vi "InitImgPath.vi"(8 "error in":errorcluster, 10 "ConfigFilePath":path, 11 "Instance":i32) -> (0 "error out":errorcluster, 2 "ImgPath":path)   [LabVIEW 2016]
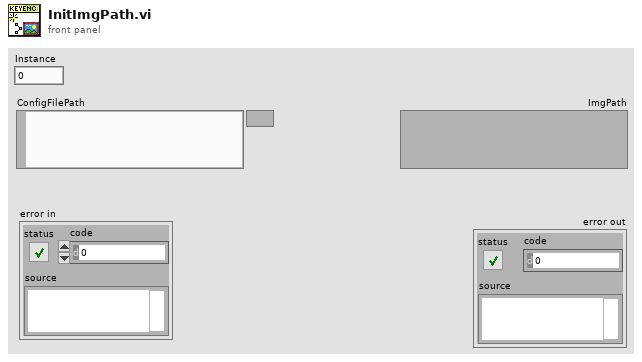
[diagram p1: front panel]
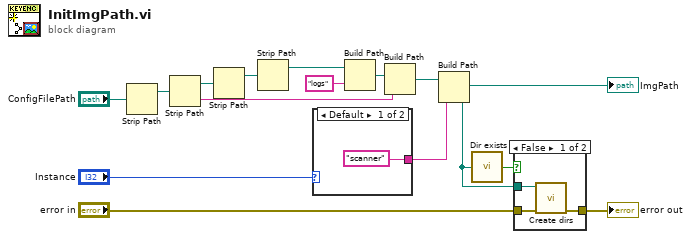
[diagram p0: block diagram]
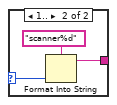
[diagram p2: hidden frame]
diagram:
  n1 = Strip Path(path="ConfigFilePath") -> (stripped path=w15:path)  [unwired: 1 out]
  n2 = Strip Path(path=w15) -> (stripped path=w14:path, name=w9:string)
  n3 = Strip Path(path=w14) -> (stripped path=w13:path)  [unwired: 1 out]
  n4 = Strip Path(path=w13) -> (stripped path=w12:path)  [unwired: 1 out]
  n5 = case shown="Default" "Instance" {
    selector: "Instance" -> [_ w17]
    tunnel: ["scanner" ("format string") w18] -> w7
    frame Default {
    }
    frame 1.. {
      n6 = Format Into String(format string="scanner%d", w17) -> (resulting string=w18:string)  [unwired: 2 in, 1 out]
    }
  }
  n7 = Build Path(base path=w12, name or relative path="logs") -> (appended path=w10:path)
  n8 = Build Path(base path=w10, name or relative path=w9) -> (appended path=w8:path)
  n9 = Build Path(base path=w8, name or relative path=w7) -> (appended path=w1:path)
  "ImgPath" <- w1
  n10 = call "Dir exists.vi"("dir path"=w1) -> ("exists?"=w2:bool)  [unwired: 4 in]
  n11 = case shown="False" w2 {
    tunnel: w1 -> [w22 _]
    tunnel: "error in" -> [w21 w23]
    tunnel: [w20 w23] -> w6
    frame False {
      n12 = call "Create dirs.vi"("error in (no error)"=w21, "deepest dir"=w22) -> ("error"=w20:errorcluster)  [unwired: 9 in]
    }
    frame True {
    }
  }
  "error out" <- w6
